vi "SENS_SWE_GRO_COUN.vi"(0 "VISA IN":refnum<visa-resource-name>, 1 "Count":i32, 5 "error in":errorcluster, 7 "Channel":i32) -> (14 "VISA Out":refnum<visa-resource-name>, 19 "error out":errorcluster)   [LabVIEW 2018, in "PNA-X.lvlib"]
doc: "SENSe<cnum>:SWEep:GROups:COUNt <num> \n(Read-Write) Sets the trigger count (groups) for the specified channel. Set trigger mode to group after setting this \ncount. \nParameters \n<cnum> Any existing channel number. If unspecified, value is set to 1 \n<num> Count (groups) number. Choose any number between: \n1 and 2e6 (1 is the same as single trigger) \nExamples SENS:SWE:GRO:COUN 10 \nsense2:sweep:groups:count 50 \nQuery Syntax SENSe<cnum>:SWEep:GROups:COUNt? \nReturn Type Numeric \nDefault 1"
uses:
  PNA-X.lvlib
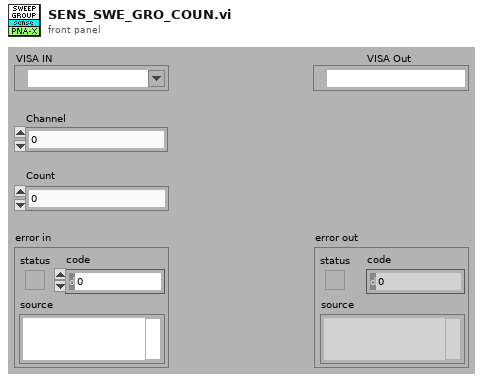
[diagram p1: front panel]
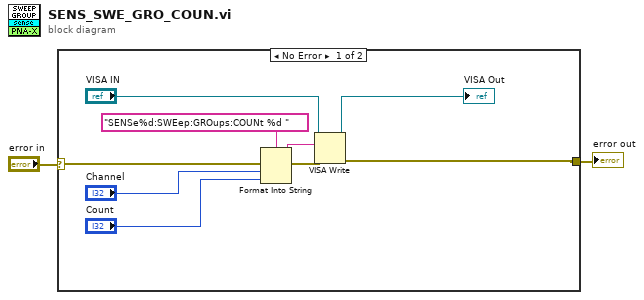
[diagram p0: block diagram]
diagram:
  n1 = case shown="No Error" "error in" {
    selector: "error in" -> [w11 w12]
    tunnel: [w6 w12] -> w1
    frame No Error {
      n2 = Format Into String(format string="SENSe%d:SWEep:GROups:COUNt %d " ("Cmdline"), error in=w11, "Channel", "Count") -> (resulting string=w9:string, error out=w10:errorcluster)  [unwired: 1 in]
      n3 = VISA Write(VISA resource name="VISA IN", write buffer=w9, error in (no error)=w10) -> (VISA resource name out=→"VISA Out":refnum<visa-resource-name>, error out=w6:errorcluster)  [unwired: 1 out]
    }
    frame Error {
    }
  }
  "error out" <- w1
